vi "poly_control_ref_from_name_self_single.vi"(8 "error in":errorcluster caption="Error in (no error)", 9 "control name":string) -> (0 "error out":errorcluster, 1 "control ref":refnum<vi>, 4 "found?":bool)   [LabVIEW 2015]
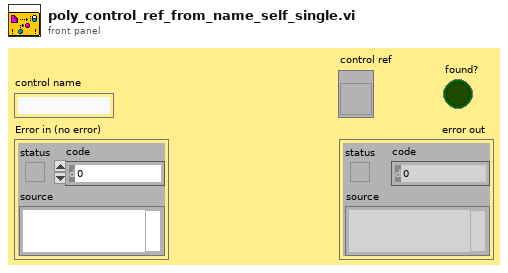
[diagram p1: front panel]
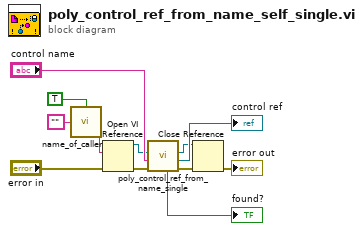
[diagram p0: block diagram]
diagram:
  n1 = call "name_of_caller.vi"("is in inlined vi? (F)"=TRUE, "name of caller in"="") -> ("name of caller out"=w11:string)  [unwired: 2 in]
  n2 = Open VI Reference(vi path=w11, error in (no error)="error in") -> (vi reference=w5:refnum<vi>, error out=w4:errorcluster)  [unwired: 4 in]
  n3 = call "poly_control_ref_from_name_single.vi"("error in (no error)"=w4, "control name"="control name", "vi ref"=w5) -> ("error out"=w2:errorcluster, "ctrl ref"=→"control ref":refnum<vi>, "vi ref dup"=w6:refnum<vi>, "found?"=→"found?":bool)  [unwired: 5 in]
  n4 = Close Reference(reference=w6, error in (no error)=w2) -> (error out=→"error out":errorcluster)
